vi "Format InstanceStatusSet_LVXML_Loop.vi"(8 "error in (no error)":errorcluster, 10 "Siblings":T2(array[cluster]), 11 "AWS_EC2 in":refnum<class "AWS_EC2.lvclass">) -> (0 "error out":errorcluster, 2 "Array":T3[](array[typedef]), 3 "AWS_EC2 out":refnum<class "AWS_EC2.lvclass">)   [LabVIEW 2014, in "AWS_EC2.lvlib" / "AWS_EC2.lvclass"]
uses:
  AWS_EC2.lvclass
  EC2 Datatypes/InstanceStatusItemType.ctl
  EC2 Datatypes/InstanceStatusEventTypeSet.ctl
  EC2 Datatypes/InstanceStatusEventType.ctl
  EC2 Datatypes/InstanceStateType.ctl
  EC2 Datatypes/InstanceStatusType.ctl
  EC2 Datatypes/InstanceStatusDetailsSetType.ctl
  lv-xml-parser/r0/trunk/VI Source/EventType.ctl
  AWS_EC2.lvlib
  lv-xml-parser/r0/trunk/VI Source/LV XML Parser.lvlib
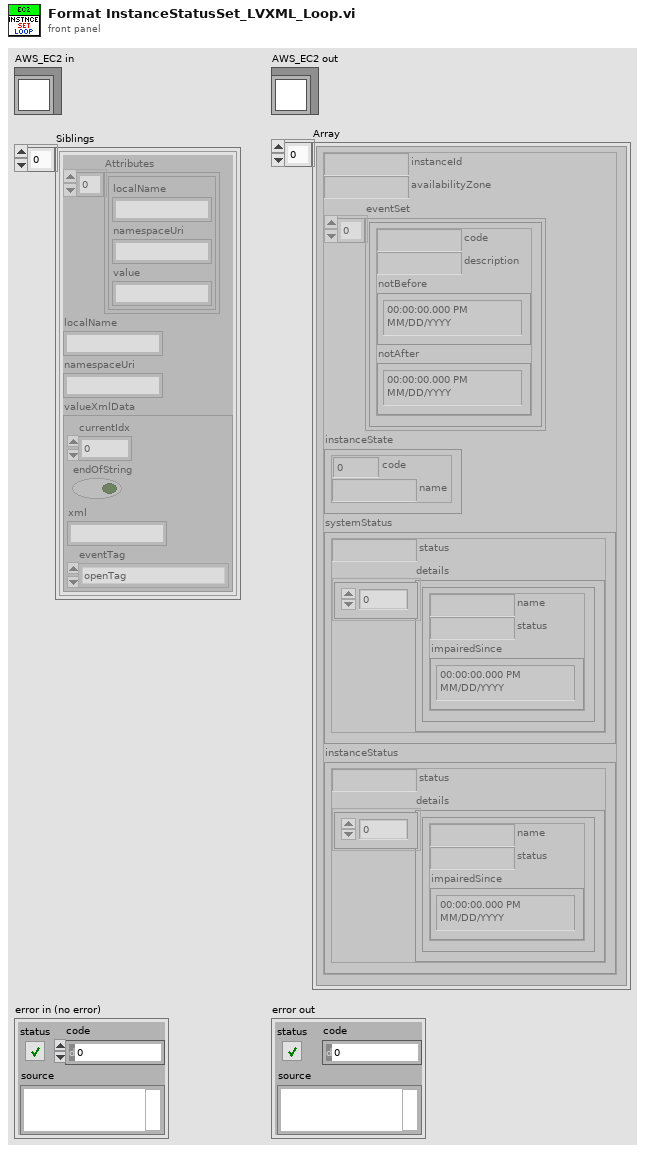
[diagram p1: front panel]
types:
  T1 = typedef "LV XML Parser.lvlib/EventType.ctl" = enum16{"openTag", "endOpenTag", "closeTag", "comment", "endComment", "endOfFile", "attribute", "startXml"}
  T2 = cluster{"Attributes":cluster{"localName":string, "namespaceUri":string, "value":string}[], "localName":string, "namespaceUri":string, "valueXmlData":cluster{"currentIdx":i32, "endOfString":bool, "xml":string, "eventTag":T1}}[]
  T3 = typedef "AWS_EC2.lvlib/InstanceStatusItemType.ctl" = cluster{"instanceId":string, "availabilityZone":string, "eventSet":T4, "instanceState":T6, "systemStatus":T7, "instanceStatus":T7}
  T4 = typedef "AWS_EC2.lvlib/InstanceStatusEventTypeSet.ctl" = T5[]
  T5 = typedef "AWS_EC2.lvlib/InstanceStatusEventType.ctl" = cluster{"code":string, "description":string, "notBefore":timestamp, "notAfter":timestamp}
  T6 = typedef "AWS_EC2.lvlib/InstanceStateType.ctl" = cluster{"code":i16, "name":string}
  T7 = typedef "AWS_EC2.lvlib/InstanceStatusType.ctl" = cluster{"status":string, "details":T8[]}
  T8 = typedef "AWS_EC2.lvlib/InstanceStatusDetailsSetType.ctl" = cluster{"name":string, "status":string, "impairedSince":timestamp}
  T9 = cluster{"Attributes":cluster{"localName":string, "namespaceUri":string, "value":string}[], "localName":string, "namespaceUri":string, "valueXmlData":cluster{"currentIdx":i32, "endOfString":bool, "xml":string, "eventTag":T1}}
  T10 = cluster{"currentIdx":i32, "endOfString":bool, "xml":string, "eventTag":T1}
  T11 = cluster{"namespaceUri":string, "localName":string}
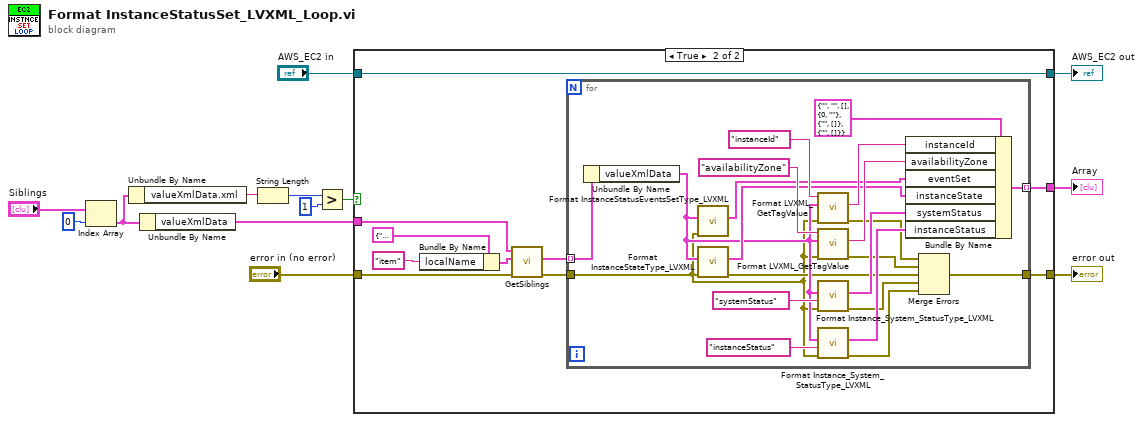
[diagram p0: block diagram]
diagram:
  n1 = Index Array(array="Siblings", index=0) -> (element=w10:T9)
  n2 = Unbundle By Name(w10) -> ("valueXmlData.xml"=w9:string)
  n3 = Unbundle By Name(w10) -> ("valueXmlData"=w8:T10)
  n4 = String Length(string=w9) -> (length=w5:i32)
  n5 = Greater?(x=w5, y=1) -> (0:w7:bool)
  n6 = case shown="True" w7 {
    tunnel: [w15 w24] -> w1
    tunnel: "error in (no error)" -> [w15 w19]
    tunnel: w8 -> [_ w18]
    tunnel: [_ w17] -> w11
    tunnel: "AWS_EC2 in" -> [w14 w16]
    tunnel: [w14 w16] -> w13
    frame False {
    }
    frame True {
      n7 = Bundle By Name(cluster=T11 {"namespaceUri"="", "localName"=""} ("limitToTag"), "localName"="item" ("Tag name")) -> (w21:T11)
      n8 = call "GetSiblings.vi"("error in (no error)"=w19, "limitToTag"=w21, "xmlData"=w18) -> ("error out"=w25:errorcluster, "Siblings"=w22:T2)  [unwired: 7 in]
      n9 = for {
        tunnel: w22 -> [w46] mode=indexing
        tunnel: [w45] -> w24
        tunnel: w25 -> [w27]
        tunnel: [w43] -> w17 mode=indexing
        n10 = Unbundle By Name(w46) -> ("valueXmlData"=w34:T10)
        n11 = call "Format InstanceStatusEventsSetType_LVXML.vi"("error in (no error)"=w27, "xmlData"=w34) -> ("InstanceStatusEventTypeSet"=w26:T4)  [unwired: 7 in, 2 out]
        n12 = call "Format InstanceStateType_LVXML.vi"("error in (no error)"=w27, "xmlData"=w34) -> ("error out"=w30:errorcluster, "InstanceStateType"=w38:T6)  [unwired: 7 in, 1 out]
        n13 = call "Format LVXML_GetTagValue.vi"("error in (no error)"=w27, "xmlDataIn"=w34, "Tag name"="instanceId") -> ("error out"=w32:errorcluster, "Value"=w41:string)  [unwired: 6 in, 1 out]
        n14 = call "Format LVXML_GetTagValue.vi"("error in (no error)"=w27, "xmlDataIn"=w34, "Tag name"="availabilityZone") -> ("error out"=w31:errorcluster, "Value"=w39:string)  [unwired: 6 in, 1 out]
        n15 = call "Format Instance_System_StatusType_LVXML.vi"("error in (no error)"=w27, "Tag name"="systemStatus", "xmlData"=w34) -> ("error out"=w29:errorcluster, "InstaneStatusType"=w37:T7)  [unwired: 6 in, 1 out]
        n16 = call "Format Instance_System_StatusType_LVXML.vi"("error in (no error)"=w27, "Tag name"="instanceStatus", "xmlData"=w34) -> ("error out"=w28:errorcluster, "InstaneStatusType"=w33:T7)  [unwired: 6 in, 1 out]
        n17 = Bundle By Name(cluster=T3 {"instanceId"="", "availabilityZone"="", "eventSet"=[], "instanceState"={"code"=0, "name"=""}, "systemStatus"={"status"="", "details"=[]}, "instanceStatus"={"status"="", "details"=[]}} ("InstanceStatusSetType"), "instanceId"=w41, "availabilityZone"=w39, "eventSet"=w26, "instanceState"=w38, "systemStatus"=w37, "instanceStatus"=w33) -> (w43:T3)
        n18 = Merge Errors(w32, w31, w30, w29, w28) -> (w45:errorcluster)
      }
    }
  }
  "AWS_EC2 out" <- w13
  "Array" <- w11
  "error out" <- w1
